vi "AM_CreateSignal.vi"() -> ()   [LabVIEW 2011]
uses:
  <vilib>/sound2/lvsound2.llb/Sound Data Format.ctl
  <vilib>/sound2/lvsound2.llb/Sampling Mode.ctl
  <vilib>/sound2/lvsound2.llb/Sound Input Read (DBL).vi
panel:
  out "Output Signal":waveform(dbl)[](array[waveform])
  out "Waveform Graph":waveform(dbl)[](graph)
  in  "Record":bool
  in  "Sound Format":T1={"sample rate (S/s)"=22050.0, "number of channels"=2, "bits per sample"=16}
  in  "Device ID":u32 format="%.0x"
  in  "Number of Samples/ch":i32=10000
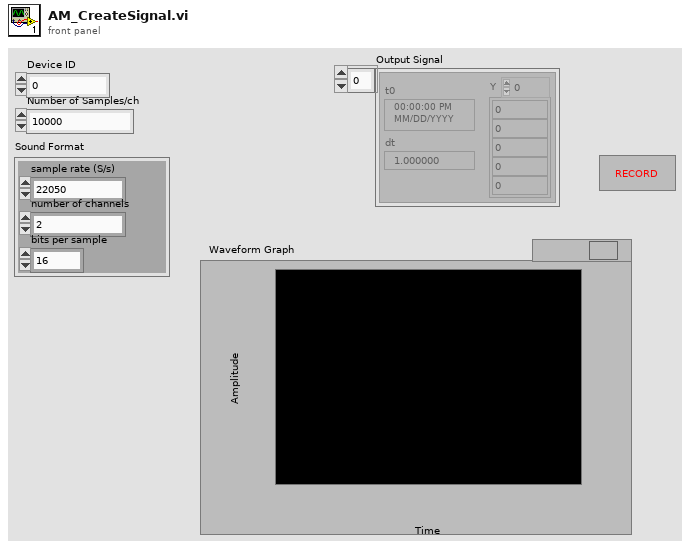
[diagram p1: front panel]
types:
  T1 = typedef "Sound Data Format.ctl" = cluster{"sample rate (S/s)":dbl, "number of channels":i32, "bits per sample":i32}
  T2 = typedef "Sampling Mode.ctl" = i32
  T3 = typedef "Sound Input Task ID.ctl" = u32
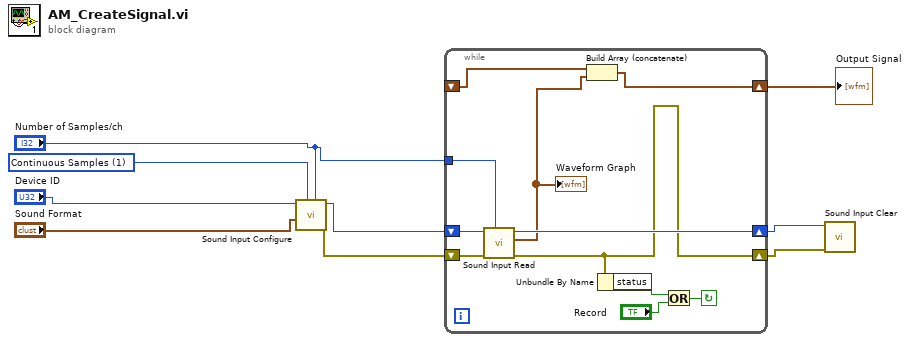
[diagram p0: block diagram]
diagram:
  w7 = T2 1 items=["Finite Samples", "Continuous Samples"] ("sample mode")
  n1 = call <vilib>:"Sound Input Configure.vi"("number of samples/ch"="Number of Samples/ch", "sample mode"=w7, "sound format"="Sound Format", "device ID"="Device ID") -> ("error out"=w5:errorcluster, "task ID"=w6:T3)  [unwired: 6 in]
  n2 = while {
    tunnel: "Number of Samples/ch" -> [w17]
    shift-right: [w18] -> w3
    shift-left: w6 -> [w19]
    shift-right: [w13] -> w2
    shift-left: w5 -> [w20]
    shift-right: [w10] -> w1
    shift-left: _ -> [w11]
    stop <- w14 continue-if-true
    n3 = call-poly <vilib>:"Sound Input Read.vi"("number of samples/ch"=w17, "error in (no error)"=w20, "task ID"=w19) -> ("error out"=w13:errorcluster, "data"=w12:waveform(dbl)[], "task ID out"=w18:T3)  [unwired: 6 in]
    "Waveform Graph" <- w12
    n4 = Build Array (concatenate)(w11, w12) -> (w10:waveform(dbl)[])
    n5 = Unbundle By Name(w13) -> ("status"=w16:bool)
    n6 = Or(x=w16, y="Record") -> (x .or. y?=w14:bool)
  }
  "Output Signal" <- w1
  n7 = call <vilib>:"Sound Input Clear.vi"("error in (no error)"=w2, "task ID"=w3) -> ()  [unwired: 9 in, 1 out]
